vi "append to kpro data array 2016.vi"(4 "Downhole Pressure Sensor":dbl format="%#_13g", 6 "Cluster in":T1, 7 "Up hole Pressure Sensor":dbl format="%.2f", 9 "Flow":dbl, 10 "Corrected Array in":dbl[][](array[numeric]), 11 "Feet of\nStainless to be\nUsed (Count) in":i32) -> (1 "IK":dbl, 2 "Array":dbl[][](array[numeric]), 3 "Cluster out 2":T1, 5 "Depth Rate":dbl format="%.2f")   [LabVIEW 2016]
uses:
  Waterloo DAQ/controls/Kpro hydraulic measurement cluster.ctl
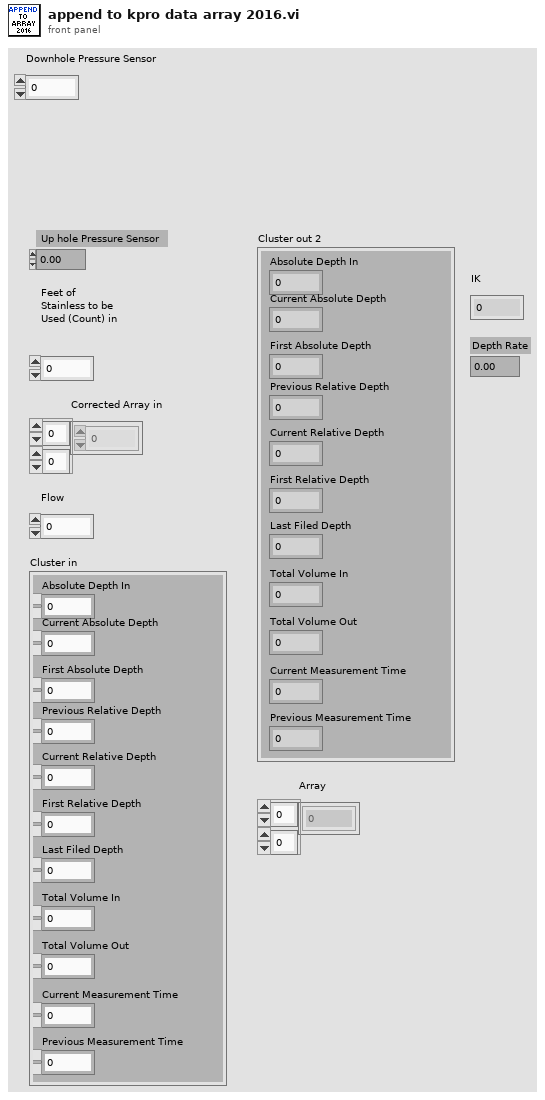
[diagram p1: front panel]
types:
  T1 = typedef "Kpro hydraulic measurement cluster.ctl" = cluster{"Absolute Depth In":dbl, "Current Absolute Depth":dbl, "First Absolute Depth":dbl, "Previous Relative Depth":dbl, "Current Relative Depth":dbl, "First Relative Depth":dbl, "Last Filed Depth":dbl, "Total Volume In":dbl, "Total Volume Out":dbl, "Current Measurement Time":dbl, "Previous Measurement Time":dbl}
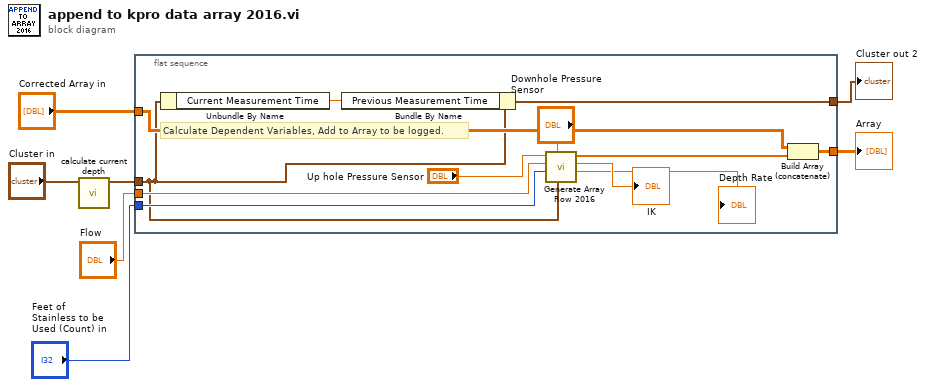
[diagram p0: block diagram]
diagram:
  n1 = call "calculate current depth.vi"("Cluster in"="Cluster in") -> ("Cluster out"=w7:T1)  [unwired: 10 in]
  n2 = flat-sequence {
    tunnel: "Corrected Array in" -> [w19]
    tunnel: [w18] -> w2
    tunnel: "Feet of\nStainless to be\nUsed (Count) in" -> [w16]
    tunnel: "Flow" -> [w15]
    tunnel: w7 -> [w13]
    tunnel: [w11] -> w5
    frame #0 {
      # "Calculate Dependent Variables, Add to Array to be logged."
      n3 = Unbundle By Name(w13) -> ("Current Measurement Time"=w12:dbl)
      n4 = Bundle By Name(cluster=w13, "Previous Measurement Time"=w12) -> (w11:T1)
      n5 = call "Generate Array Row 2016.vi"("Cluster"=w13, "Downhole Pressure Sensor"="Downhole Pressure Sensor", "Feet of\nStainless to be\nUsed (Count)"=w16, "Flow"=w15, "In line Pressure Sensor"="Up hole Pressure Sensor") -> ("Depth Rate"=→"Depth Rate":dbl, "IK"=→"IK":dbl, "Array"=w17:dbl[])  [unwired: 4 in]
      n6 = Build Array (concatenate)(w19, w17) -> (w18:dbl[][])
    }
  }
  "Cluster out 2" <- w5
  "Array" <- w2
